vi "TR_Load_TDMS_parameters.vi"(0 "TDMS track path in":path, 11 "error in (no error)":errorcluster) -> (3 "File version":string, 4 "Basic settings":T17={"Vert. offset"=0.0, "Hor. offset"=0.0, "Bridge swap"=FALSE, "Twisted neck"=FALSE, "Cage diam."=325, "Magn.rot."=0, "Acq. speed"=0.0} {"Acq. speed" format="%_5f fps"; "Magn.rot." min=-180 max=180 step=1 format="%.0d°"; "Cage diam." format="%.0u mm"; "Hor. offset" format="%#_1f mm"; "Vert. offset" format="%#_1f mm"}, 6 "1st frame HW timestamp":i32, 8 "Full settings":T1={"Defaults"={"Default User"=0.0, "VISA Resource Name "="Tracker", "Histogram parameters"={"max"=300.0, "min"=0.0, "# bins"=10, "threshold"=8.0, "thr. type"=enum."higher accepted"}}, "Recording and saving"={"Researcher name"="Researcher", "Name prefix"="Track", "Data post-processing"={"Filter type"=enum."Savitzky-Golay", "Length"=31, "Order"=3}, "Stop at"=0.0, "\"Stop at\" enabled"=FALSE, "Default save folder path"=path "", "Acquisition FPS"=enum."Max"}, "Geometry"={"Cage diameter, mm"=180, "Starting angle MIDFIELD"=0, "Starting angle BORDER"=0, "Radius, mm CENTER"=30, "Radius, mm MIDFIELD"=75, "N segments MIDFIELD"=2, "N segments BORDER"=4, "R-gap, mm"=0.0, "Bridge swap"=FALSE, "Bridge H. offset"=0.0, "Bridge V. offset"=0.0, "Twisted neck"=FALSE, "Alt. magn. orientation"=FALSE, "Sensor board size"=enum."Small"}, "IO parameters"={"IO general config."=12, "IO 1 configuration"=1, "IO 2 configuration"=1, "IO 3 configuration"=0, "IO 4 configuration"=0, "Activate ext. RS-232"=0, "IO inversion config."=0, "Sync capability"=1}, "Conditions presets array"=[{"Enabled"=FALSE, "Name"="", "Specifier(s)"=[], "Response"={"Response type"=enum."Air puff", "TTL port"=enum."Port 1", "TTL pulse length, ms"=0.0}, "Has been set"=FALSE}, {"Enabled"=FALSE, "Name"="", "Specifier(s)"=[], "Response"={"Response type"=enum."Air puff", "TTL port"=enum."Port 1", "TTL pulse length, ms"=0.0}, "Has been set"=FALSE}, {"Enabled"=FALSE, "Name"="", "Specifier(s)"=[], "Response"={"Response type"=enum."Air puff", "TTL port"=enum."Port 1", "TTL pulse length, ms"=0.0}, "Has been set"=FALSE}, {"Enabled"=FALSE, "Name"="", "Specifier(s)"=[], "Response"={"Response type"=enum."Air puff", "TTL port"=enum."Port 1", "TTL pulse length, ms"=0.0}, "Has been set"=FALSE}, {"Enabled"=FALSE, "Name"="", "Specifier(s)"=[], "Response"={"Response type"=enum."Air puff", "TTL port"=enum."Port 1", "TTL pulse length, ms"=0.0}, "Has been set"=FALSE}, {"Enabled"=FALSE, "Name"="", "Specifier(s)"=[], "Response"={"Response type"=enum."Air puff", "TTL port"=enum."Port 1", "TTL pulse length, ms"=0.0}, "Has been set"=FALSE}, {"Enabled"=FALSE, "Name"="", "Specifier(s)"=[], "Response"={"Response type"=enum."Air puff", "TTL port"=enum."Port 1", "TTL pulse length, ms"=0.0}, "Has been set"=FALSE}, {"Enabled"=FALSE, "Name"="", "Specifier(s)"=[], "Response"={"Response type"=enum."Air puff", "TTL port"=enum."Port 1", "TTL pulse length, ms"=0.0}, "Has been set"=FALSE}, {"Enabled"=FALSE, "Name"="", "Specifier(s)"=[], "Response"={"Response type"=enum."Air puff", "TTL port"=enum."Port 1", "TTL pulse length, ms"=0.0}, "Has been set"=FALSE}, {"Enabled"=FALSE, "Name"="", "Specifier(s)"=[], "Response"={"Response type"=enum."Air puff", "TTL port"=enum."Port 1", "TTL pulse length, ms"=0.0}, "Has been set"=FALSE}, {"Enabled"=FALSE, "Name"="", "Specifier(s)"=[], "Response"={"Response type"=enum."Air puff", "TTL port"=enum."Port 1", "TTL pulse length, ms"=0.0}, "Has been set"=FALSE}, {"Enabled"=FALSE, "Name"="", "Specifier(s)"=[], "Response"={"Response type"=enum."Air puff", "TTL port"=enum."Port 1", "TTL pulse length, ms"=0.0}, "Has been set"=FALSE}, {"Enabled"=FALSE, "Name"="", "Specifier(s)"=[], "Response"={"Response type"=enum."Air puff", "TTL port"=enum."Port 1", "TTL pulse length, ms"=0.0}, "Has been set"=FALSE}, {"Enabled"=FALSE, "Name"="", "Specifier(s)"=[], "Response"={"Response type"=enum."Air puff", "TTL port"=enum."Port 1", "TTL pulse length, ms"=0.0}, "Has been set"=FALSE}], "Calibration parameters"={"Timing calibration sw/hw"=1.0, "True FPS"=80.0, "True frame time, s"=0.0125, "Disp. calibration info"=[]}, "Settings loaded OK"=FALSE} {"Calibration parameters"."True frame time, s" format="%.10g"; "Calibration parameters"."Disp. calibration info"."Speed, µl per ms" format="%.3g"; "Calibration parameters"."True FPS" format="%.10g"; "Calibration parameters"."Timing calibration sw/hw" format="%.10g"; "Conditions presets array"."Specifier(s)"."Validity criteria(s)"."Validity value" min=0.0 step=0.1 format="%.2g"; "Conditions presets array"."Specifier(s)"."Value" step=1.0 format="%#.2g"; "Recording and saving"."Data post-processing"."Order" min=3 max=11 step=2; "Recording and saving"."Data post-processing"."Length" min=5 max=301 step=2; "Geometry"."Cage diameter, mm" scale=0.0..340.0}, 10 "1st frame SW timestamp":timestamp, 14 "TDMS track path out":path, 15 "error out":errorcluster)   [LabVIEW 2018, in "Tracks Repair.lvlib"]
uses:
  Libraries/Tracks Repair/Tracks Repair.lvlib
  Controls/CTL_Basic_cage_settings.ctl
  Controls/CTL_Settings_cluster.ctl
  Controls/CTL_Histogram_parameters.ctl
  Controls/CTL_Filter_selector.ctl
  Controls/CTL_Acquisition_speed_selector.ctl
  Controls/CTL_Segmented_plot_parameters.ctl
  Controls/CTL_IO_params_cluster.ctl
  Controls/CTL_Conditions_Array.ctl
  Controls/CTL_Conditions_Cluster.ctl
  Controls/CTL_Condition_type.ctl
  Controls/CTL_Comparison_type.ctl
  Controls/CTL_Validity_check_criteria.ctl
  Controls/CTL_Response_info.ctl
  Controls/CTL_Condition_response_type.ctl
  Controls/CTL_Reponse_port_info.ctl
  Controls/CTL_Calibration_parameters.ctl
  Controls/CTL_Dispenser_calibration_info.ctl
  Tracker.lvlib
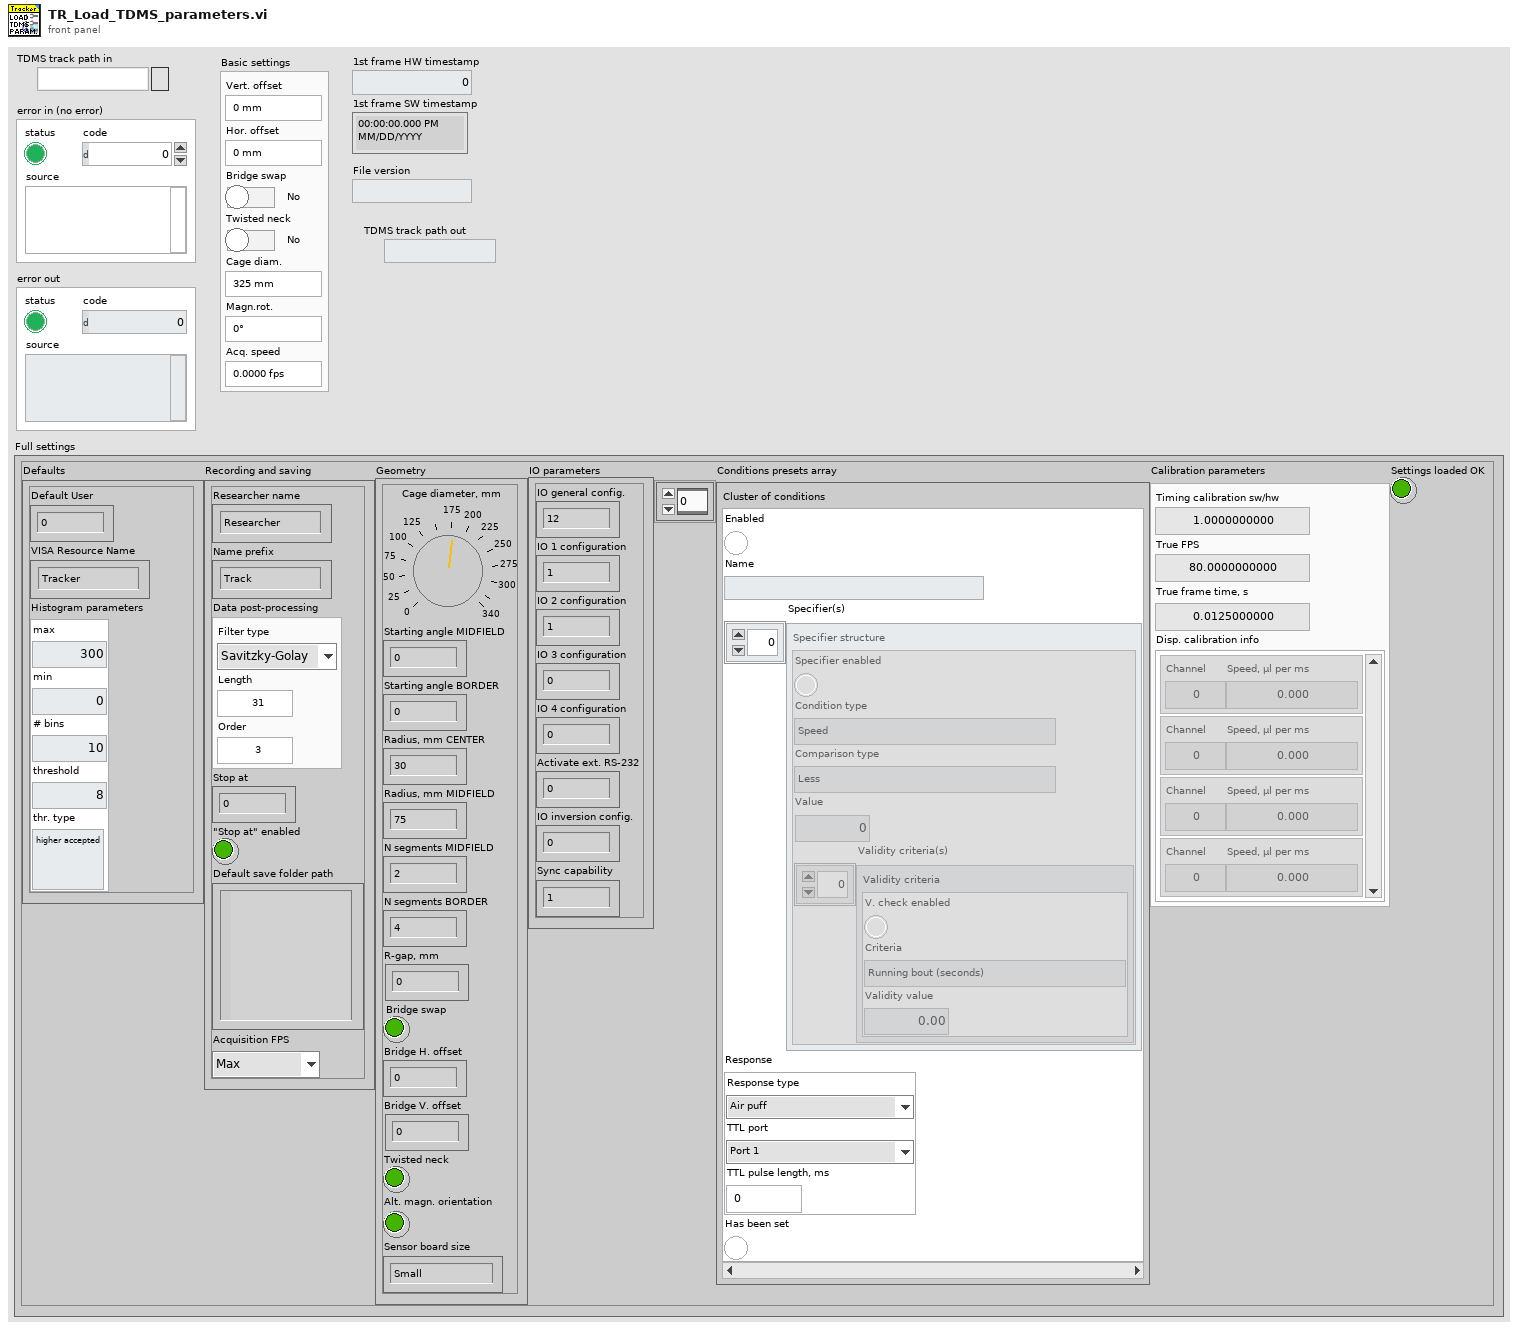
[diagram p1: front panel]
types:
  T1 = typedef "Tracker.lvlib/CTL_Settings_cluster.ctl" = cluster{"Defaults":cluster{"Default User":dbl, "VISA Resource Name ":string, "Histogram parameters":T2}, "Recording and saving":cluster{"Researcher name":string, "Name prefix":string, "Data post-processing":T3, "Stop at":dbl, "\"Stop at\" enabled":bool, "Default save folder path":path, "Acquisition FPS":T4}, "Geometry":T5, "IO parameters":T6, "Conditions presets array":T7, "Calibration parameters":T15, "Settings loaded OK":bool}
  T2 = typedef "Tracker.lvlib/CTL_Histogram_parameters.ctl" = cluster{"max":dbl, "min":dbl, "# bins":i32, "threshold":dbl, "thr. type":enum16{"higher accepted", "lower accepted"}}
  T3 = typedef "Tracker.lvlib/CTL_Filter_selector.ctl" = cluster{"Filter type":enum16{"None", "Savitzky-Golay"}, "Length":i32, "Order":i32}
  T4 = typedef "Tracker.lvlib/CTL_Acquisition_speed_selector.ctl" = enum16{"Max", "Optimal", "Eco"}
  T5 = typedef "Tracker.lvlib/CTL_Segmented_plot_parameters.ctl" = cluster{"Cage diameter, mm":u16, "Starting angle MIDFIELD":i16, "Starting angle BORDER":i16, "Radius, mm CENTER":u16, "Radius, mm MIDFIELD":u16, "N segments MIDFIELD":u8, "N segments BORDER":u8, "R-gap, mm":sgl, "Bridge swap":bool, "Bridge H. offset":sgl, "Bridge V. offset":sgl, "Twisted neck":bool, "Alt. magn. orientation":bool, "Sensor board size":enum16{"Small", "Large"}}
  T6 = typedef "Tracker.lvlib/CTL_IO_params_cluster.ctl" = cluster{"IO general config.":u16, "IO 1 configuration":u16, "IO 2 configuration":u16, "IO 3 configuration":u16, "IO 4 configuration":u16, "Activate ext. RS-232":u16, "IO inversion config.":u16, "Sync capability":u8}
  T7 = typedef "Tracker.lvlib/CTL_Conditions_Array.ctl" = T8[]
  T8 = typedef "Tracker.lvlib/CTL_Conditions_Cluster.ctl" = cluster{"Enabled":bool, "Name":string, "Specifier(s)":cluster{"Specifier enabled":bool, "Condition type":T9, "Comparison type":T10, "Value":dbl, "Validity criteria(s)":cluster{"V. check enabled":bool, "Criteria":T11, "Validity value":dbl}[]}[], "Response":T12, "Has been set":bool}
  T9 = typedef "Tracker.lvlib/CTL_Condition_type.ctl" = enum16{"Speed", "Zone", "Angle to wall"}
  T10 = typedef "Tracker.lvlib/CTL_Comparison_type.ctl" = enum16{"Less", "Less or Equal", "Equal", "Greater or Equal", "Greater", "Not Equal"}
  T11 = typedef "Tracker.lvlib/CTL_Validity_check_criteria.ctl" = enum16{"Running bout (seconds)", "Running bout (meters)"}
  T12 = typedef "Tracker.lvlib/CTL_Response_info.ctl" = cluster{"Response type":T13, "TTL port":T14, "TTL pulse length, ms":dbl}
  T13 = typedef "Tracker.lvlib/CTL_Condition_response_type.ctl" = enum16{"None", "Air puff", "Liquid reward"}
  T14 = typedef "Tracker.lvlib/CTL_Reponse_port_info.ctl" = enum16{"Port 1", "Port 2", "Port 3", "Port 4"}
  T15 = typedef "Tracker.lvlib/CTL_Calibration_parameters.ctl" = cluster{"Timing calibration sw/hw":dbl, "True FPS":dbl, "True frame time, s":dbl, "Disp. calibration info":T16}
  T16 = typedef "Tracker.lvlib/CTL_Dispenser_calibration_info.ctl" = cluster{"Channel":u8, "Speed, µl per ms":dbl}[]
  T17 = typedef "Tracker.lvlib/CTL_Basic_cage_settings.ctl" = cluster{"Vert. offset":dbl, "Hor. offset":dbl, "Bridge swap":bool, "Twisted neck":bool, "Cage diam.":i32, "Magn.rot.":i32, "Acq. speed":dbl}
  T18 = enum16{"big-endian, network order", "native, host order", "little-endian"}
  T19 = enum16{"open", "open or create", "create or replace", "create", "open (read-only)"}
  T20 = cluster{"Absolute timestamp (DBL)":dbl[], "Relative timestamp (DBL)":dbl[], "Zones normalized allocation array":dbl[][], "Coordinates and speed":dbl[][], "Current zone and TTLs":u8[][], "Acquisition settings cluster out":cluster{"Researcher name":string, "N segments MIDFIELD":u8, "N segments BORDER":u8, "Radius, mm CENTER":u16, "Radius, mm MIDFIELD":u16, "Starting angle MIDFIELD":i16, "Starting angle BORDER":i16, "Cage diameter, mm":u16, "Bridge swap":bool, "Bridge V. offset":sgl, "Twisted neck":bool, "Offset H.":sgl, "Name prefix":string, "Stop at":dbl, "\"Stop at\" enabled":bool, "Settings loaded OK":bool}, "Stimulus presets array":cluster{"Event type":u16, "Time, s":sgl, "Stimulus, s":sgl, "Set/Clear":bool, "TTL out":u16, "Stim. has been set":bool}[]}
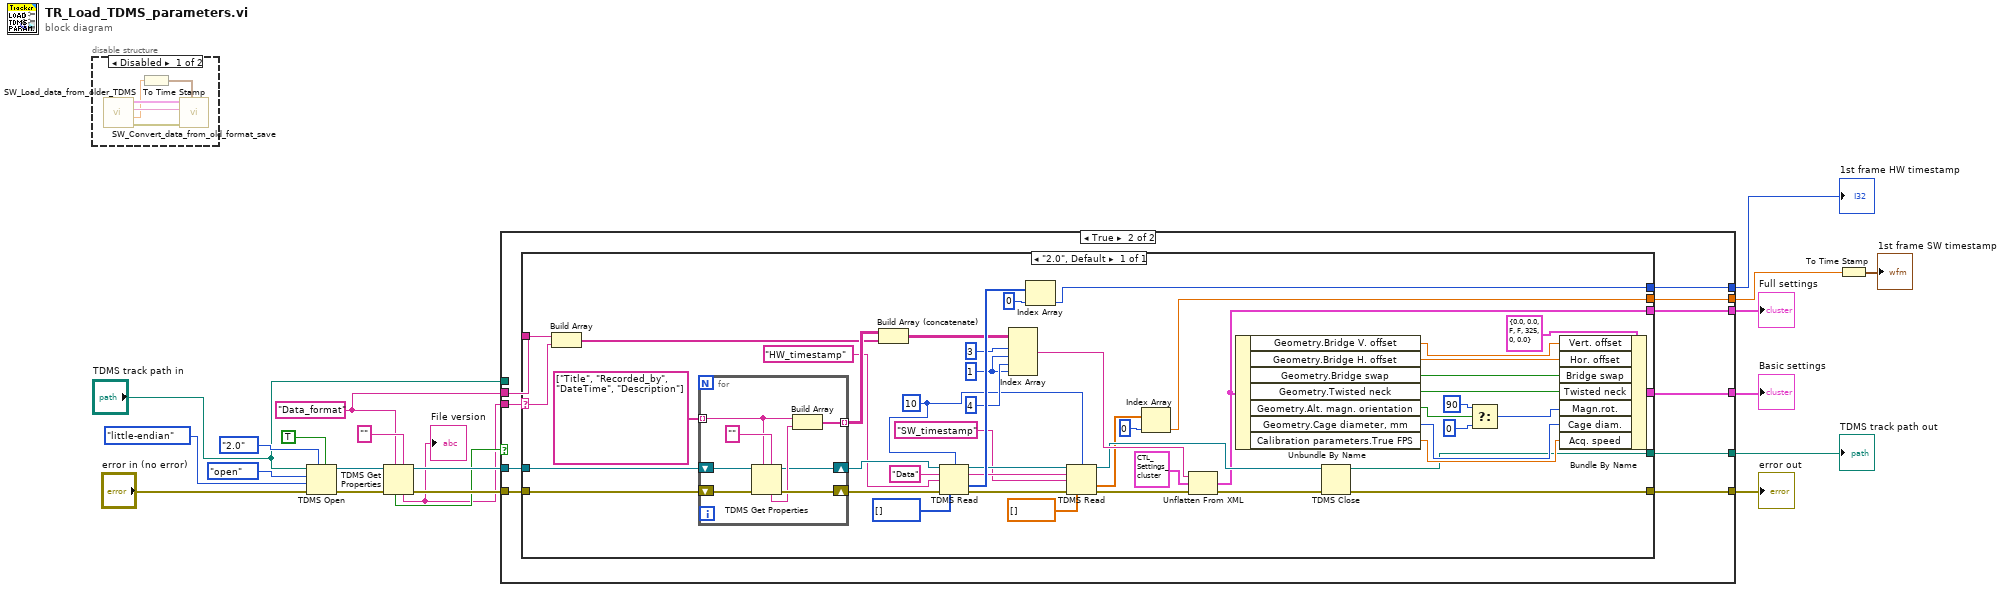
[diagram p0: block diagram]
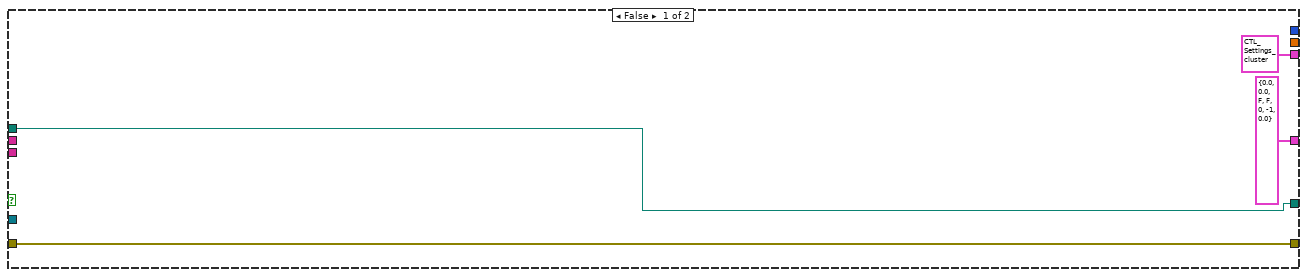
[diagram p3: hidden frame]
diagram:
  w8 = "Data_format"
  n1 = disable-structure shown="Disabled" {
    frame Disabled {
      n2 = call "SW_Load_data_from_older_TDMS.vi"() -> ("error out"=w25:errorcluster, "Start time"=w23:dbl, "Author's name"=w24:string, "Loaded data"=w26:T20)  [unwired: 6 in, 2 out]
      n3 = To Time Stamp(1:w23) -> (0:w22:timestamp)
      n4 = call "SW_Convert_data_from_old_format_save.vi"("Time Stamp in"=w22, "error in (no error)"=w25, "Researcher name"=w24, "Loaded data in"=w26) -> ()  [unwired: 6 in, 2 out]
    }
    frame Enabled {
    }
  }
  n5 = TDMS Open(5:TRUE ("create index file? (T)"), 7:enum16{"1.0", "2.0"}."2.0" ("file format version (2.0)"), 8:"error in (no error)", 9:T18."little-endian" ("byte order (2:little-endian)"), 10:T19."open" ("operation (0:open)"), 11:"TDMS track path in") -> (0:w14:errorcluster, 3:w15:refnum<k34>)  [unwired: 1 in]
  n6 = TDMS Get Properties(5:"", 7:w8, 8:w14, 11:w15) -> (0:w13:errorcluster, 3:w12:refnum<k34>, 4:w10:string, 6:w11:bool)  [unwired: 2 in, 2 out]
  "File version" <- w10
  n7 = case shown="True" w11 {
    tunnel: w13 -> [w30 w40]
    tunnel: w12 -> [_ w39]
    tunnel: w10 -> [_ w38]
    tunnel: [w30 w37] -> w9
    tunnel: w8 -> [_ w36]
    tunnel: [T17 {"Vert. offset"=0.0, "Hor. offset"=0.0, "Bridge swap"=FALSE, "Twisted neck"=FALSE, "Cage diam."=0, "Magn.rot."=-1, "Acq. speed"=0.0} ("Settings") w35] -> w7
    tunnel: [_ w34] -> w5
    tunnel: [_ w33] -> w6
    tunnel: [w28 w32] -> w3
    tunnel: "TDMS track path in" -> [w28 _]
    tunnel: [T1 {"Defaults"={"Default User"=-1.0, "VISA Resource Name "="Tracker", "Histogram parameters"={"max"=300.0, "min"=0.0, "# bins"=10, "threshold"=8.0, "thr. type"=enum."higher accepted"}}, "Recording and saving"={"Researcher name"="Researcher", "Name prefix"="Track", "Data post-processing"={"Filter type"=enum."Savitzky-Golay", "Length"=31, "Order"=3}, "Stop at"=0.0, "\"Stop at\" enabled"=FALSE, "Default save folder path"=path "", "Acquisition FPS"=enum."Max"}, "Geometry"={"Cage diameter, mm"=0, "Starting angle MIDFIELD"=0, "Starting angle BORDER"=0, "Radius, mm CENTER"=30, "Radius, mm MIDFIELD"=75, "N segments MIDFIELD"=2, "N segments BORDER"=4, "R-gap, mm"=0.0, "Bridge swap"=FALSE, "Bridge H. offset"=0.0, "Bridge V. offset"=0.0, "Twisted neck"=FALSE, "Alt. magn. orientation"=FALSE, "Sensor board size"=enum."Small"}, "IO parameters"={"IO general config."=12, "IO 1 configuration"=1, "IO 2 configuration"=1, "IO 3 configuration"=0, "IO 4 configuration"=0, "Activate ext. RS-232"=0, "IO inversion config."=0, "Sync capability"=1}, "Conditions presets array"=[{"Enabled"=FALSE, "Name"="", "Specifier(s)"=[], "Response"={"Response type"=enum."Air puff", "TTL port"=enum."Port 1", "TTL pulse length, ms"=0.0}, "Has been set"=FALSE}, {"Enabled"=FALSE, "Name"="", "Specifier(s)"=[], "Response"={"Response type"=enum."Air puff", "TTL port"=enum."Port 1", "TTL pulse length, ms"=0.0}, "Has been set"=FALSE}, {"Enabled"=FALSE, "Name"="", "Specifier(s)"=[], "Response"={"Response type"=enum."Air puff", "TTL port"=enum."Port 1", "TTL pulse length, ms"=0.0}, "Has been set"=FALSE}, {"Enabled"=FALSE, "Name"="", "Specifier(s)"=[], "Response"={"Response type"=enum."Air puff", "TTL port"=enum."Port 1", "TTL pulse length, ms"=0.0}, "Has been set"=FALSE}, {"Enabled"=FALSE, "Name"="", "Specifier(s)"=[], "Response"={"Response type"=enum."Air puff", "TTL port"=enum."Port 1", "TTL pulse length, ms"=0.0}, "Has been set"=FALSE}, {"Enabled"=FALSE, "Name"="", "Specifier(s)"=[], "Response"={"Response type"=enum."Air puff", "TTL port"=enum."Port 1", "TTL pulse length, ms"=0.0}, "Has been set"=FALSE}, {"Enabled"=FALSE, "Name"="", "Specifier(s)"=[], "Response"={"Response type"=enum."Air puff", "TTL port"=enum."Port 1", "TTL pulse length, ms"=0.0}, "Has been set"=FALSE}, {"Enabled"=FALSE, "Name"="", "Specifier(s)"=[], "Response"={"Response type"=enum."Air puff", "TTL port"=enum."Port 1", "TTL pulse length, ms"=0.0}, "Has been set"=FALSE}, {"Enabled"=FALSE, "Name"="", "Specifier(s)"=[], "Response"={"Response type"=enum."Air puff", "TTL port"=enum."Port 1", "TTL pulse length, ms"=0.0}, "Has been set"=FALSE}, {"Enabled"=FALSE, "Name"="", "Specifier(s)"=[], "Response"={"Response type"=enum."Air puff", "TTL port"=enum."Port 1", "TTL pulse length, ms"=0.0}, "Has been set"=FALSE}, {"Enabled"=FALSE, "Name"="", "Specifier(s)"=[], "Response"={"Response type"=enum."Air puff", "TTL port"=enum."Port 1", "TTL pulse length, ms"=0.0}, "Has been set"=FALSE}, {"Enabled"=FALSE, "Name"="", "Specifier(s)"=[], "Response"={"Response type"=enum."Air puff", "TTL port"=enum."Port 1", "TTL pulse length, ms"=0.0}, "Has been set"=FALSE}, {"Enabled"=FALSE, "Name"="", "Specifier(s)"=[], "Response"={"Response type"=enum."Air puff", "TTL port"=enum."Port 1", "TTL pulse length, ms"=0.0}, "Has been set"=FALSE}, {"Enabled"=FALSE, "Name"="", "Specifier(s)"=[], "Response"={"Response type"=enum."Air puff", "TTL port"=enum."Port 1", "TTL pulse length, ms"=0.0}, "Has been set"=FALSE}], "Calibration parameters"={"Timing calibration sw/hw"=1.0, "True FPS"=80.0, "True frame time, s"=0.0125, "Disp. calibration info"=[]}, "Settings loaded OK"=FALSE} ("Settings cluster") w31] -> w1
    frame False {
    }
    frame True {
      n8 = case shown="\"2.0\", Default" w38 {
        selector: w38 -> [w81]
        tunnel: w40 -> [w83]
        tunnel: w39 -> [w82]
        tunnel: [w68] -> w37
        tunnel: w36 -> [w79]
        tunnel: [w57] -> w35
        tunnel: [w56] -> w34
        tunnel: [w44] -> w33
        tunnel: [w42] -> w32
        tunnel: [w41] -> w31
        frame "2.0", Default {
          w73 = 1 ("disabled index (col)")
          w48 = i64 10 ("count (-1: all)")
          n9 = Build Array(w79, w81) -> (w80:string[])
          n10 = for {
            tunnel: string[] ["Title", "Recorded_by", "DateTime", "Description"] ("property names") -> [w92] mode=indexing
            tunnel: [w90] -> w84 mode=indexing
            shift-right: [w89] -> w85
            shift-left: w82 -> [w95]
            shift-right: [w93] -> w86
            shift-left: w83 -> [w96]
            n11 = TDMS Get Properties(5:"", 7:w92, 8:w96, 11:w95) -> (0:w93:errorcluster, 3:w89:refnum<k34>, 4:w91:string)  [unwired: 2 in, 3 out]
            n12 = Build Array(w92, w91) -> (w90:string[])
          }
          n13 = Build Array (concatenate)(w84, w80) -> (w70:string[][])
          n14 = TDMS Read(0:w85, 2:w48, 5:"Data" ("group name in"), 7:"HW_timestamp", 11:w86, 12:i32[] []) -> (4:w53:refnum<k34>, 6:w54:string, 10:w77:i32[], 15:w51:errorcluster)  [unwired: 2 in, 2 out]
          n15 = Index Array(array=w70, index (row) #1=3 ("index (row)"), index (col) #1=w73, index (row) #2=4 ("index (row)"), index (col) #2=w73) -> (element #1=w72:string)  [unwired: 1 out]
          n16 = Index Array(array=w77, index=0 ("index (row)")) -> (element=w56:i32)
          n17 = TDMS Read(0:w53, 2:w48, 5:w54, 7:"SW_timestamp", 11:w51, 12:dbl[] []) -> (4:w52:refnum<k34>, 10:w49:dbl[], 15:w50:errorcluster)  [unwired: 2 in, 3 out]
          n18 = Index Array(array=w49, index=0 ("index (row)")) -> (element=w44:dbl)
          n19 = Unflatten From XML(xml string=w72, type=T1 {"Defaults"={"Default User"=0.0, "VISA Resource Name "="Tracker", "Histogram parameters"={"max"=300.0, "min"=0.0, "# bins"=10, "threshold"=8.0, "thr. type"=enum."higher accepted"}}, "Recording and saving"={"Researcher name"="Researcher", "Name prefix"="Track", "Data post-processing"={"Filter type"=enum."Savitzky-Golay", "Length"=31, "Order"=3}, "Stop at"=0.0, "\"Stop at\" enabled"=FALSE, "Default save folder path"=path "", "Acquisition FPS"=enum."Max"}, "Geometry"={"Cage diameter, mm"=180, "Starting angle MIDFIELD"=0, "Starting angle BORDER"=0, "Radius, mm CENTER"=30, "Radius, mm MIDFIELD"=75, "N segments MIDFIELD"=2, "N segments BORDER"=4, "R-gap, mm"=0.0, "Bridge swap"=FALSE, "Bridge H. offset"=0.0, "Bridge V. offset"=0.0, "Twisted neck"=FALSE, "Alt. magn. orientation"=FALSE, "Sensor board size"=enum."Small"}, "IO parameters"={"IO general config."=12, "IO 1 configuration"=1, "IO 2 configuration"=1, "IO 3 configuration"=0, "IO 4 configuration"=0, "Activate ext. RS-232"=0, "IO inversion config."=0, "Sync capability"=1}, "Conditions presets array"=[{"Enabled"=FALSE, "Name"="", "Specifier(s)"=[], "Response"={"Response type"=enum."Air puff", "TTL port"=enum."Port 1", "TTL pulse length, ms"=0.0}, "Has been set"=FALSE}, {"Enabled"=FALSE, "Name"="", "Specifier(s)"=[], "Response"={"Response type"=enum."Air puff", "TTL port"=enum."Port 1", "TTL pulse length, ms"=0.0}, "Has been set"=FALSE}, {"Enabled"=FALSE, "Name"="", "Specifier(s)"=[], "Response"={"Response type"=enum."Air puff", "TTL port"=enum."Port 1", "TTL pulse length, ms"=0.0}, "Has been set"=FALSE}, {"Enabled"=FALSE, "Name"="", "Specifier(s)"=[], "Response"={"Response type"=enum."Air puff", "TTL port"=enum."Port 1", "TTL pulse length, ms"=0.0}, "Has been set"=FALSE}, {"Enabled"=FALSE, "Name"="", "Specifier(s)"=[], "Response"={"Response type"=enum."Air puff", "TTL port"=enum."Port 1", "TTL pulse length, ms"=0.0}, "Has been set"=FALSE}, {"Enabled"=FALSE, "Name"="", "Specifier(s)"=[], "Response"={"Response type"=enum."Air puff", "TTL port"=enum."Port 1", "TTL pulse length, ms"=0.0}, "Has been set"=FALSE}, {"Enabled"=FALSE, "Name"="", "Specifier(s)"=[], "Response"={"Response type"=enum."Air puff", "TTL port"=enum."Port 1", "TTL pulse length, ms"=0.0}, "Has been set"=FALSE}, {"Enabled"=FALSE, "Name"="", "Specifier(s)"=[], "Response"={"Response type"=enum."Air puff", "TTL port"=enum."Port 1", "TTL pulse length, ms"=0.0}, "Has been set"=FALSE}, {"Enabled"=FALSE, "Name"="", "Specifier(s)"=[], "Response"={"Response type"=enum."Air puff", "TTL port"=enum."Port 1", "TTL pulse length, ms"=0.0}, "Has been set"=FALSE}, {"Enabled"=FALSE, "Name"="", "Specifier(s)"=[], "Response"={"Response type"=enum."Air puff", "TTL port"=enum."Port 1", "TTL pulse length, ms"=0.0}, "Has been set"=FALSE}, {"Enabled"=FALSE, "Name"="", "Specifier(s)"=[], "Response"={"Response type"=enum."Air puff", "TTL port"=enum."Port 1", "TTL pulse length, ms"=0.0}, "Has been set"=FALSE}, {"Enabled"=FALSE, "Name"="", "Specifier(s)"=[], "Response"={"Response type"=enum."Air puff", "TTL port"=enum."Port 1", "TTL pulse length, ms"=0.0}, "Has been set"=FALSE}, {"Enabled"=FALSE, "Name"="", "Specifier(s)"=[], "Response"={"Response type"=enum."Air puff", "TTL port"=enum."Port 1", "TTL pulse length, ms"=0.0}, "Has been set"=FALSE}, {"Enabled"=FALSE, "Name"="", "Specifier(s)"=[], "Response"={"Response type"=enum."Air puff", "TTL port"=enum."Port 1", "TTL pulse length, ms"=0.0}, "Has been set"=FALSE}], "Calibration parameters"={"Timing calibration sw/hw"=1.0, "True FPS"=80.0, "True frame time, s"=0.0125, "Disp. calibration info"=[]}, "Settings loaded OK"=FALSE} ("Settings cluster"), error in (no error)=w50) -> (value=w41:T1, error out=w69:errorcluster)
          n20 = Unbundle By Name(w41) -> ("Geometry.Bridge V. offset"=w66:sgl, "Geometry.Bridge H. offset"=w65:sgl, "Geometry.Bridge swap"=w64:bool, "Geometry.Twisted neck"=w63:bool, "Geometry.Alt. magn. orientation"=w62:bool, "Geometry.Cage diameter, mm"=w58:u16, "Calibration parameters.True FPS"=w43:dbl)
          n21 = TDMS Close(8:w69, 11:w52) -> (0:w68:errorcluster, 3:w42:path)
          n22 = Select(t=90 ("Magn.rot."), s=w62, f=0 ("Magn.rot.")) -> (s? t:f=w59:i32)
          n23 = Bundle By Name(cluster=T17 {"Vert. offset"=0.0, "Hor. offset"=0.0, "Bridge swap"=FALSE, "Twisted neck"=FALSE, "Cage diam."=325, "Magn.rot."=0, "Acq. speed"=0.0} ("Settings"), "Vert. offset"=w66, "Hor. offset"=w65, "Bridge swap"=w64, "Twisted neck"=w63, "Magn.rot."=w59, "Cage diam."=w58, "Acq. speed"=w43) -> (w57:T17)
        }
      }
    }
  }
  "error out" <- w9
  "Basic settings" <- w7
  "1st frame HW timestamp" <- w5
  "TDMS track path out" <- w3
  "Full settings" <- w1
  n24 = To Time Stamp(1:w6) -> (0:→"1st frame SW timestamp":timestamp)
